vi "Download Multiple Files.vi"(6 "timeout (ms)":i32=30000, 8 "error in":errorcluster, 10 "file specifications":T1[](array[typedef]), 11 "session in":refnum<class "Session.lvclass">) -> (0 "error out":errorcluster, 3 "session out":refnum<class "Session.lvclass">)   [LabVIEW 2020, in "NI_SFTP.lvlib"]
doc: "Downloads multiple files."
uses:
  <vilib>/net/SFTP/NI_SFTP.lvlib
  <vilib>/net/SFTP/Session/Session.lvclass
  <vilib>/net/SFTP/API/Support/File Specification.ctl
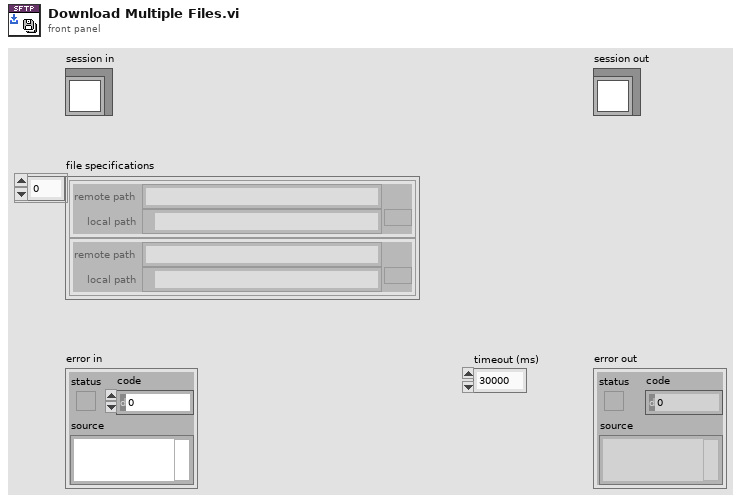
[diagram p1: front panel]
types:
  T1 = typedef "NI_SFTP.lvlib/File Specification.ctl" = cluster{"remote path":string, "local path":path}
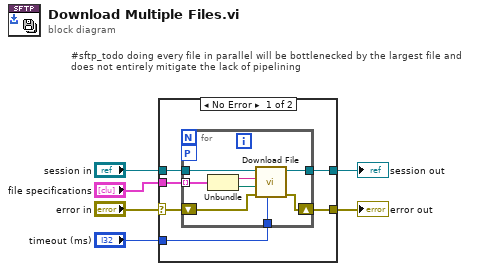
[diagram p0: block diagram]
diagram:
  # "#sftp_todo doing every file in parallel will be bottlenecked by the largest file and does not entirely mitigate the lack of pipelining"
  n1 = case shown="No Error" "error in" {
    selector: "error in" -> [w8 w22]
    tunnel: [w9 w22] -> w6
    tunnel: [w11 w21] -> w4
    tunnel: "session in" -> [w12 w21]
    tunnel: "timeout (ms)" -> [w10 _]
    tunnel: "file specifications" -> [w7 _]
    frame No Error {
      n2 = for {
        workers-P: _ -> [_]
        tunnel: w12 -> [w20]
        tunnel: [w18] -> w11
        tunnel: w10 -> [w16]
        shift-right: [w17] -> w9
        shift-left: w8 -> [w19]
        tunnel: w7 -> [w15] mode=indexing
        n3 = Unbundle(w15) -> ("remote path"=w14:string, "local path"=w13:path)
        n4 = call <vilib>:"Download File.vi"("timeout (ms)"=w16, "error in"=w19, "local path"=w13, "remote path"=w14, "session in"=w20) -> ("error out"=w17:errorcluster, "session out"=w18:refnum<class "Session.lvclass">)  [unwired: 5 in]
      }
    }
    frame Error {
    }
  }
  "error out" <- w6
  "session out" <- w4
